vi "Read outer terminal.vi"(9 "Tunnel in":refnum<class "Tunnel.lvclass">) -> (3 "Tunnel out":refnum<class "Tunnel.lvclass">, 4 "outer terminal":refnum<class "Terminal.lvclass">)   [LabVIEW 2014, in "Raspberry Pi Compatible Compiler for LabVIEW.lvlib" / "Tunnel.lvclass"]
uses:
  Tunnel.lvclass
  Terminal/Terminal.lvclass
  Tunnel.lvclass/Tunnel.ctl
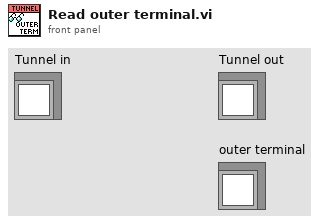
[diagram p1: front panel]
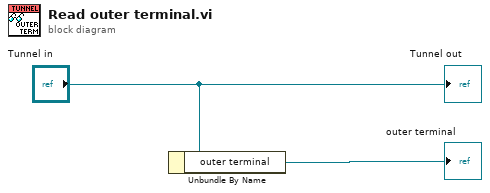
[diagram p0: block diagram]
diagram:
  n1 = Unbundle By Name("Tunnel in") -> ("outer terminal"=→"outer terminal":refnum<class "Terminal.lvclass">)
  "Tunnel out" <- "Tunnel in"
